vi "Data.vi"(11 "Pop Up Msg in":refnum<class "Pop Up Msg.lvclass">) -> ()   [LabVIEW 2021, in "Pop Up.lvlib" / "Pop Up Msg.lvclass"]
uses:
  Pop Up Msg.lvclass
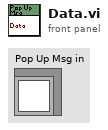
[diagram p1: front panel]
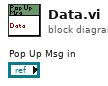
[diagram p0: block diagram]
diagram:
